vi "Initialize_VI.vi"() -> ()   [LabVIEW 2021]
panel:
  in  "Inputs":cluster{dbl, dbl, dbl}
  in  "Select initailize":T1(ring)=enum.""
  in  "error constant":errorcluster
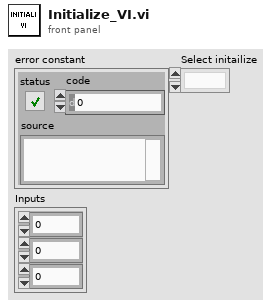
[diagram p1: front panel]
types:
  T1 = enum16{"Initialize_Leser", "Iintiailize_Motor", ""}
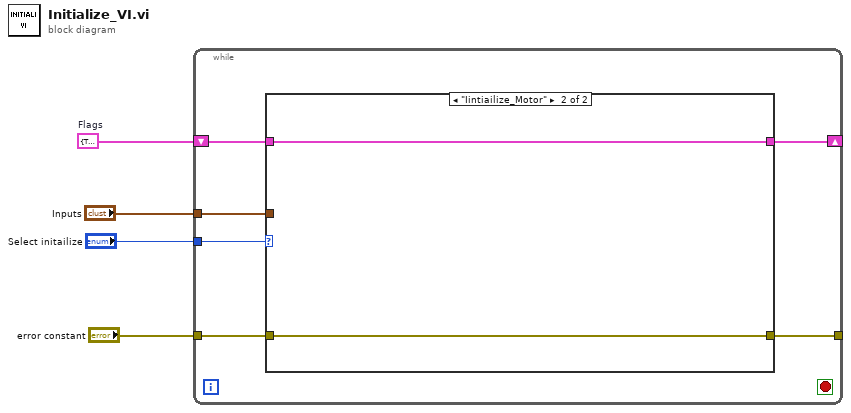
[diagram p0: block diagram]
diagram:
  w4 = cluster{bool, bool, bool, bool} {TRUE, TRUE, TRUE, TRUE}  # Flags
  n1 = while {
    shift-right: [w9] -> _
    shift-left: w4 -> [w10]
    tunnel: "error constant" -> [w7]
    tunnel: [w8] -> _
    tunnel: "Select initailize" -> [w6]
    tunnel: "Inputs" -> [w5]
    stop <- _ stop-if-true
    n2 = case shown="\"Iintiailize_Motor\"" w6 {
      tunnel: w10 -> [w11 w14]
      tunnel: [w11 w14] -> w9
      tunnel: [w12 w13] -> w8
      tunnel: w7 -> [w12 w13]
      tunnel: w5 -> [_ _]
      frame "Initialize_Leser", Default {
      }
      frame "Iintiailize_Motor" {
      }
    }
  }
